vi "PopulateExposureTime.vi"(10 "Exposure Time":refnum<vi>, 11 ".NET Refnum in":refnum<k24>) -> ()   [LabVIEW 2018]
uses:
  D:/SVN/PM/sdk/AppSamples/LabVIEWSamples/trunk/Release/2018/Dependencies/PVCamNET.dll
  Dependencies/PVCamNET.dll
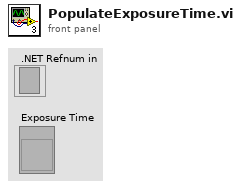
[diagram p1: front panel]
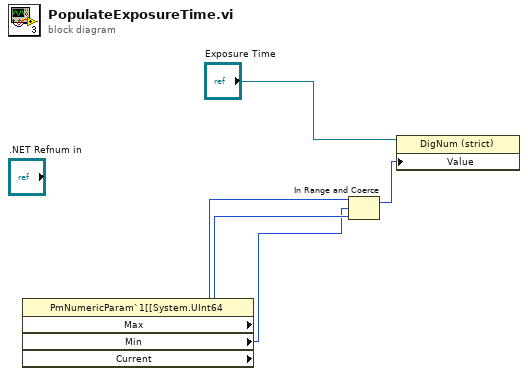
[diagram p0: block diagram]
diagram:
  n1 = property class="PmNumericParam`1[[System.UInt64"() -> ("Max"=w3:u64, "Min"=w1:u64, "Current"=w2:u64)  [unwired: 2 in, 2 out]
  n2 = In Range and Coerce(upper limit=w3, x=w1, lower limit=w2) -> (coerced(x)=w5:u64)  [unwired: 1 out]
  n3 = property class="DigNum (strict)"(reference="Exposure Time", "Value"=w5) -> ()  [unwired: 1 in, 2 out]
